vi "Read Limit Test.vi"(0 "VISA resource name":refnum<visa-resource-name>, 5 "Measurement Type (6: Phase Noise)":u16(ring)=6 items=["AM Noise"=1, "Baseband Noise"=2, "Freq/Power"=3, "Spectrum"=4, "Transient"=5, "Phase Noise"=6, "User"=7], 11 "error in (no error)":errorcluster, 12 "Maximum Time (10000 ms)":u32=10000) -> (1 "Trace 1 Result":enum16{"Pass", "Fail", ""}(ring)=enum."", 2 "Trace 2 Result":enum16{"Pass", "Fail", ""}(ring)=enum."", 3 "Trace 3 Result":enum16{"Pass", "Fail", ""}(ring)=enum."", 4 "VISA resource name out":refnum<visa-resource-name>, 6 "Trace 4 Result":enum16{"Pass", "Fail", ""}(ring)=enum."", 8 "Trace 5 Result":enum16{"Pass", "Fail", ""}(ring)=enum."", 10 "Trace 6 Result":enum16{"Pass", "Fail", ""}(ring)=enum."", 13 "Trace 8 Result":enum16{"Pass", "Fail", ""}(ring)=enum."", 14 "Trace 7 Result":enum16{"Pass", "Fail", ""}(ring)=enum."", 15 "error out":errorcluster)   [LabVIEW 2011, in "Agilent E5052X.lvlib"]
doc: "Reads the limit line test results for all traces and all kinds of measurements.\n\n<b>Note: </b> \n\nUse the \"Clear-Load Limit Line\" utility VI to load a user specified limit line. Use the \"Configure Limit Test\" VI to enable the limit line and change other settings. If \"Enable Limit Line\" control in the \"Configure Limit Test\" VI is not enabled, the test will always pass."
uses:
  Agilent E5052X.lvlib
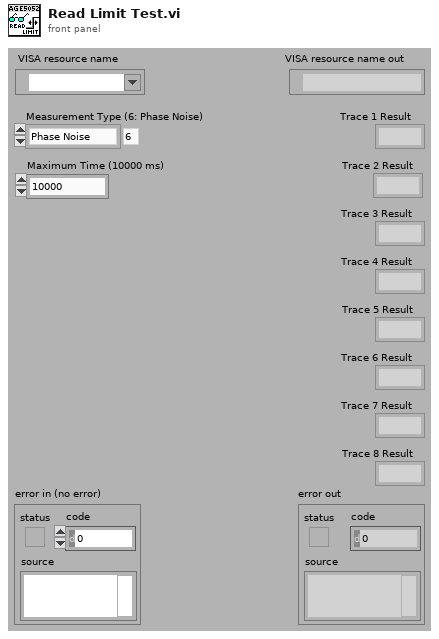
[diagram p1: front panel]
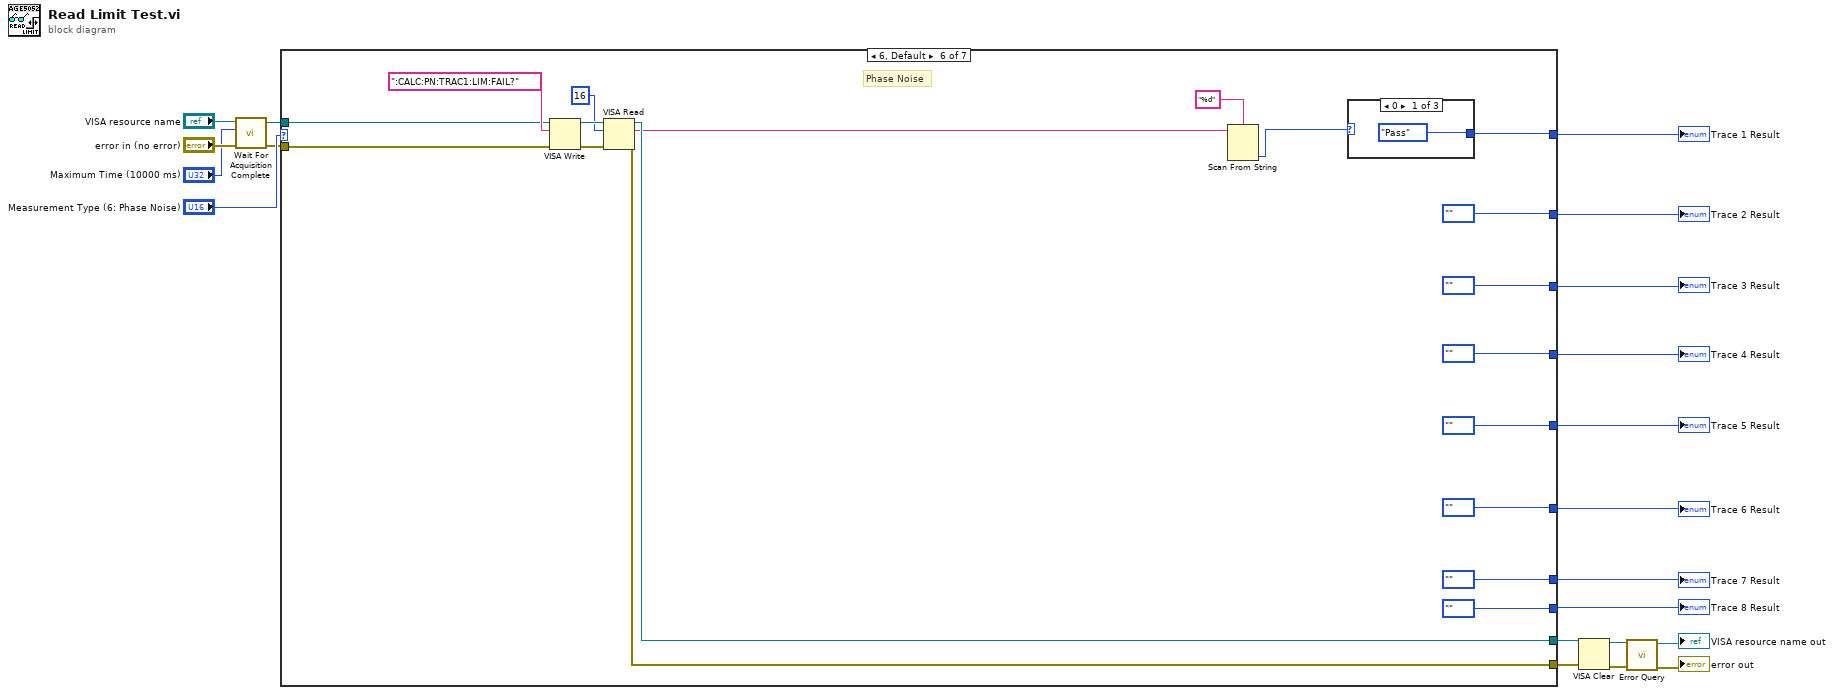
[diagram p0: block diagram]
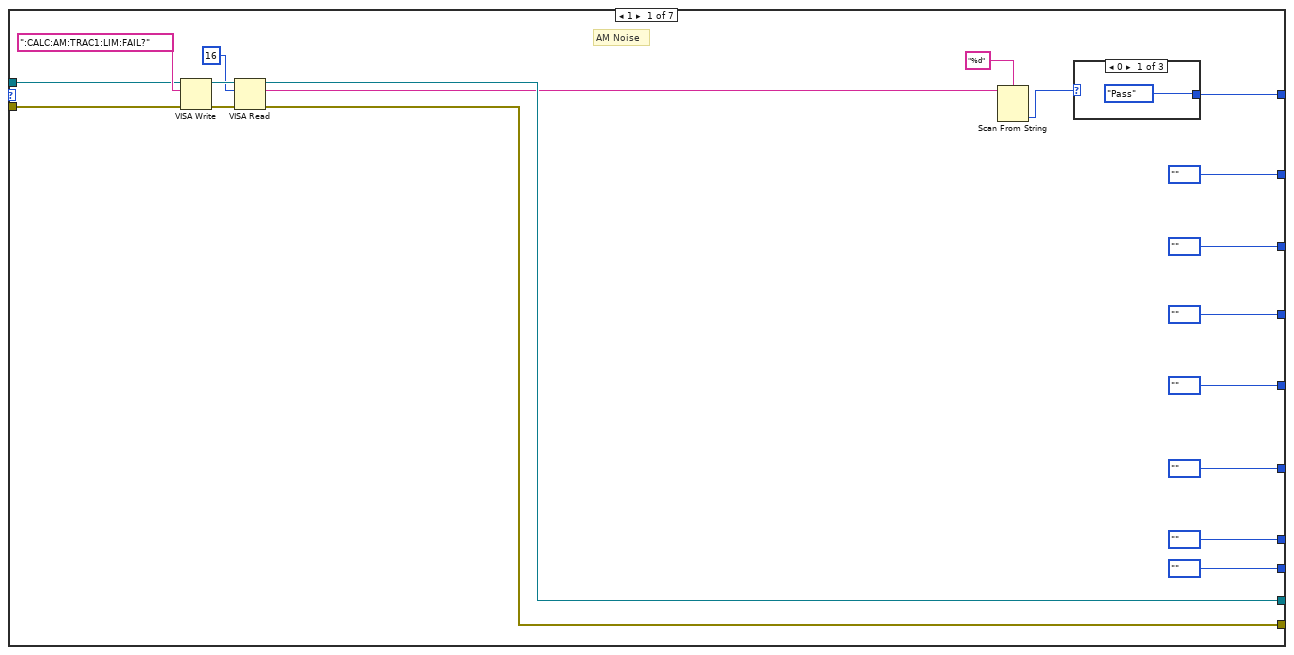
[diagram p2: hidden frame]
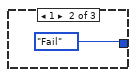
[diagram p3: hidden frame]
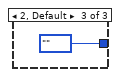
[diagram p4: hidden frame]
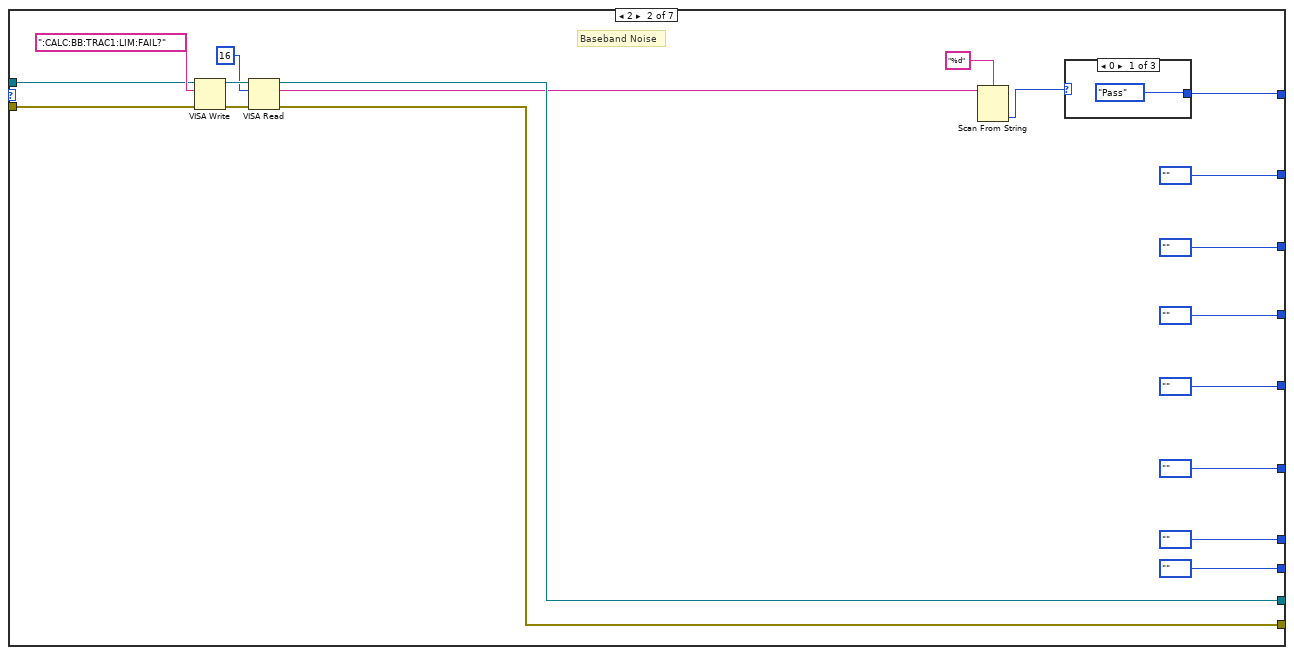
[diagram p5: hidden frame]
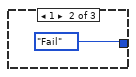
[diagram p6: hidden frame]
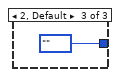
[diagram p7: hidden frame]
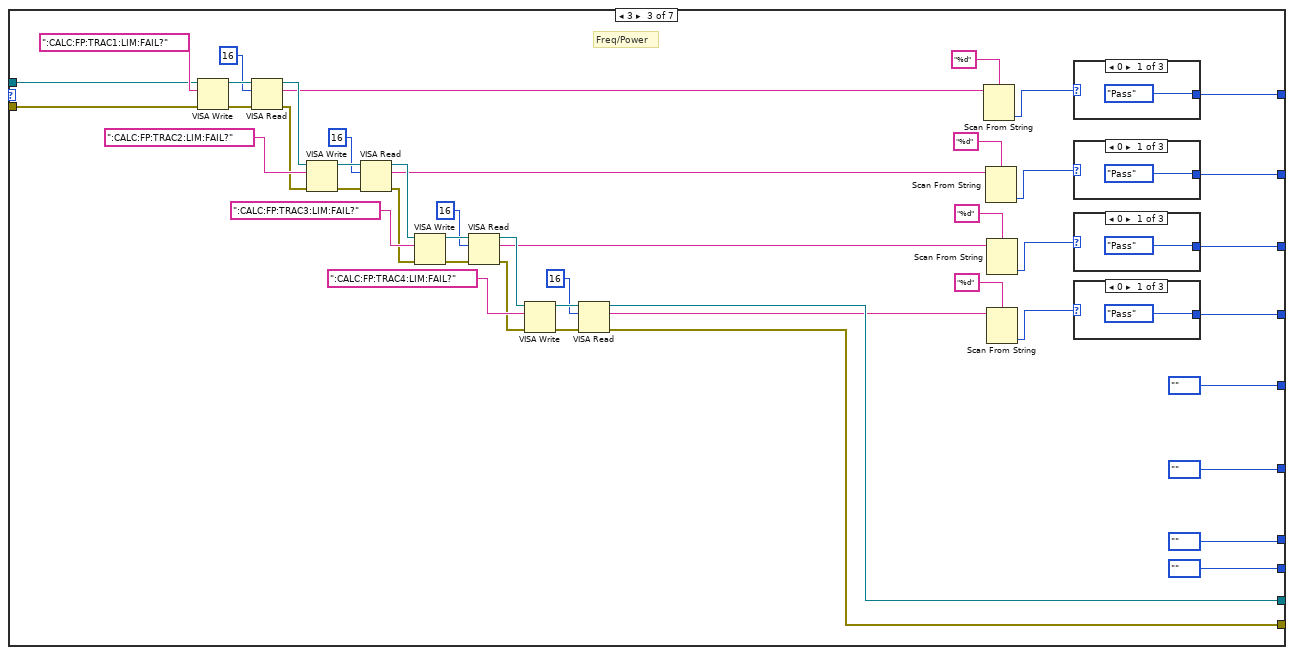
[diagram p8: hidden frame]
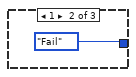
[diagram p9: hidden frame]
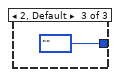
[diagram p10: hidden frame]
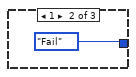
[diagram p11: hidden frame]
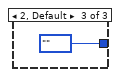
[diagram p12: hidden frame]
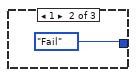
[diagram p13: hidden frame]
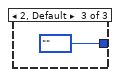
[diagram p14: hidden frame]
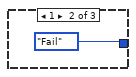
[diagram p15: hidden frame]
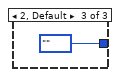
[diagram p16: hidden frame]
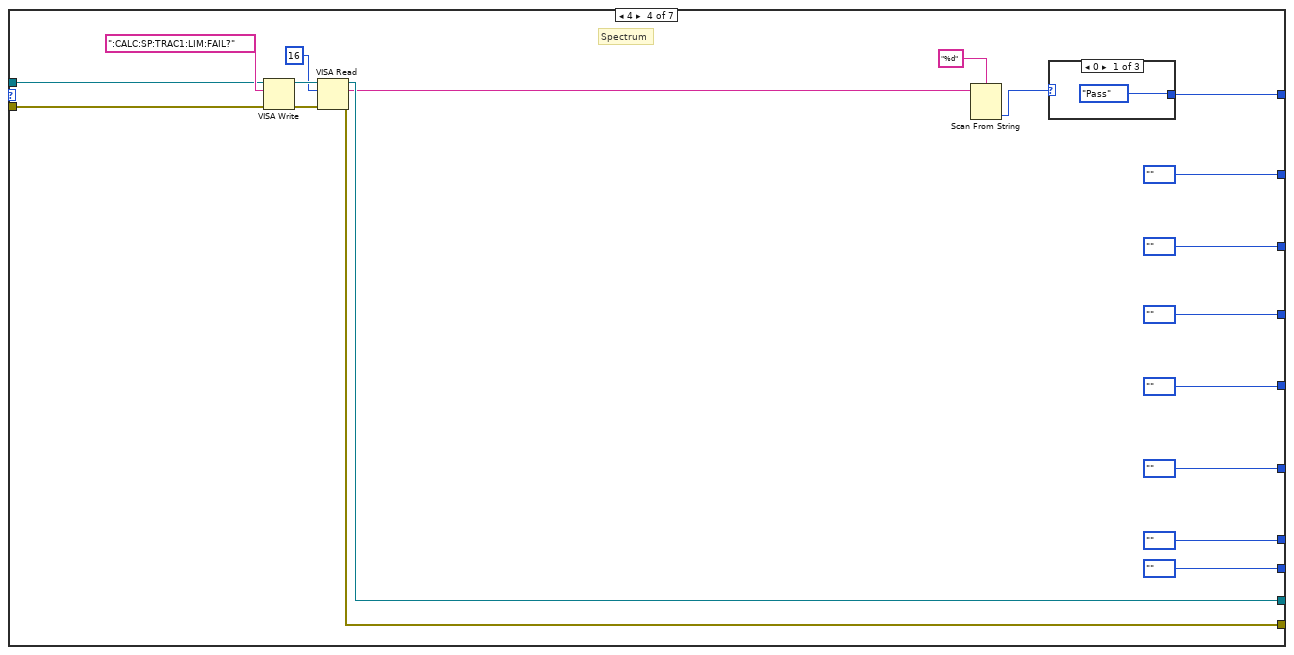
[diagram p17: hidden frame]
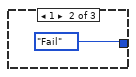
[diagram p18: hidden frame]
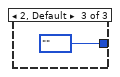
[diagram p19: hidden frame]
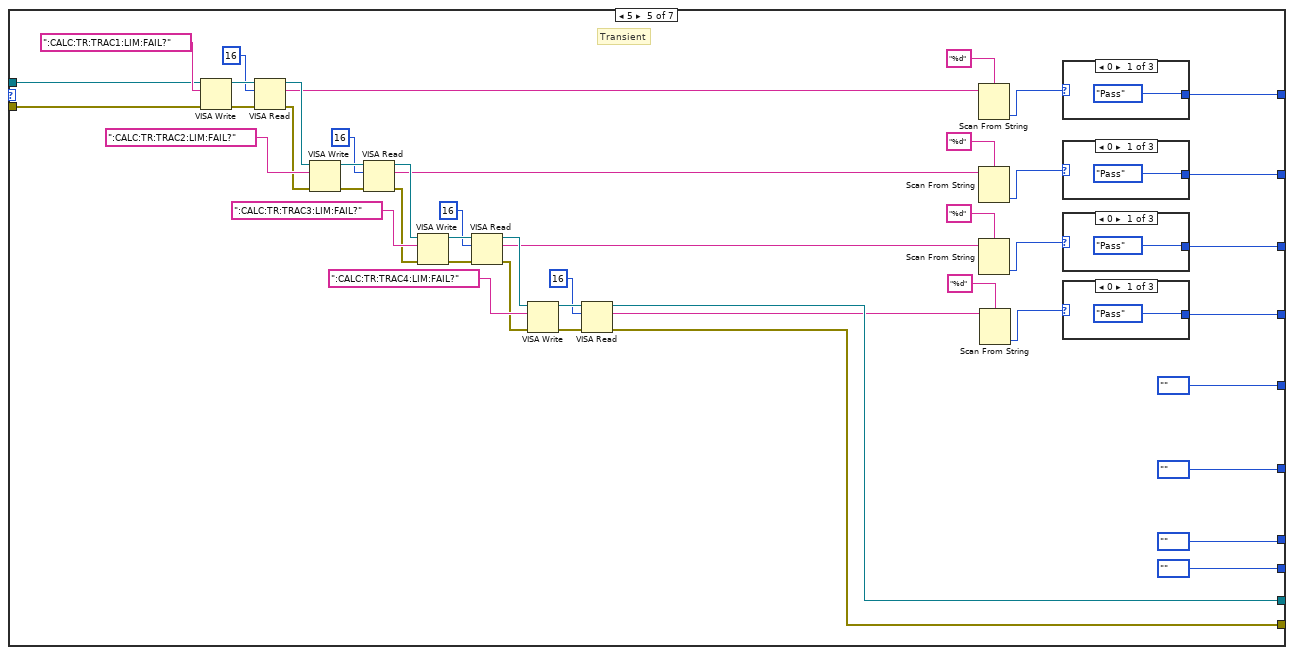
[diagram p20: hidden frame]
diagram:
  n1 = call "Wait For Acquisition Complete.vi"("error in (no error)"="error in (no error)", "Maximum Time (10000)"="Maximum Time (10000 ms)", "VISA resource name"="VISA resource name") -> ("error out"=w6:errorcluster, "VISA resource name out"=w7:refnum<visa-resource-name>)  [unwired: 7 in]
  n2 = case shown="6, Default" "Measurement Type (6: Phase Noise)" {
    tunnel: w7 -> [w35 w57 w106 w137 w168 w217 w284]
    tunnel: w6 -> [w34 w56 w105 w136 w167 w216 w283]
    tunnel: [w33 w55 w86 w135 w166 w215 w258] -> w12
    tunnel: [w32 w54 w85 w134 w165 w214 w257] -> w11
    tunnel: [w31 w53 w84 w133 w164 w213 w256] -> w20
    tunnel: [enum16{"Pass", "Fail", ""}."" ("Trace 1 Result") enum16{"Pass", "Fail", ""}."" ("Trace 1 Result") w83 enum16{"Pass", "Fail", ""}."" ("Trace 1 Result") w163 enum16{"Pass", "Fail", ""}."" ("Trace 1 Result") w255] -> w19
    tunnel: [enum16{"Pass", "Fail", ""}."" ("Trace 1 Result") enum16{"Pass", "Fail", ""}."" ("Trace 1 Result") w82 enum16{"Pass", "Fail", ""}."" ("Trace 1 Result") w162 enum16{"Pass", "Fail", ""}."" ("Trace 1 Result") w254] -> w18
    tunnel: [enum16{"Pass", "Fail", ""}."" ("Trace 1 Result") enum16{"Pass", "Fail", ""}."" ("Trace 1 Result") w81 enum16{"Pass", "Fail", ""}."" ("Trace 1 Result") w161 enum16{"Pass", "Fail", ""}."" ("Trace 1 Result") w253] -> w17
    tunnel: [enum16{"Pass", "Fail", ""}."" ("Trace 1 Result") enum16{"Pass", "Fail", ""}."" ("Trace 1 Result") enum16{"Pass", "Fail", ""}."" ("Trace 1 Result") enum16{"Pass", "Fail", ""}."" ("Trace 1 Result") enum16{"Pass", "Fail", ""}."" ("Trace 1 Result") enum16{"Pass", "Fail", ""}."" ("Trace 1 Result") w249] -> w16
    tunnel: [enum16{"Pass", "Fail", ""}."" ("Trace 1 Result") enum16{"Pass", "Fail", ""}."" ("Trace 1 Result") enum16{"Pass", "Fail", ""}."" ("Trace 1 Result") enum16{"Pass", "Fail", ""}."" ("Trace 1 Result") enum16{"Pass", "Fail", ""}."" ("Trace 1 Result") enum16{"Pass", "Fail", ""}."" ("Trace 1 Result") w250] -> w15
    tunnel: [enum16{"Pass", "Fail", ""}."" ("Trace 1 Result") enum16{"Pass", "Fail", ""}."" ("Trace 1 Result") enum16{"Pass", "Fail", ""}."" ("Trace 1 Result") enum16{"Pass", "Fail", ""}."" ("Trace 1 Result") enum16{"Pass", "Fail", ""}."" ("Trace 1 Result") enum16{"Pass", "Fail", ""}."" ("Trace 1 Result") w251] -> w14
    tunnel: [enum16{"Pass", "Fail", ""}."" ("Trace 1 Result") enum16{"Pass", "Fail", ""}."" ("Trace 1 Result") enum16{"Pass", "Fail", ""}."" ("Trace 1 Result") enum16{"Pass", "Fail", ""}."" ("Trace 1 Result") enum16{"Pass", "Fail", ""}."" ("Trace 1 Result") enum16{"Pass", "Fail", ""}."" ("Trace 1 Result") w252] -> w13
    frame 1 {
      # "AM Noise"
      n3 = VISA Write(VISA resource name=w35, write buffer=":CALC:AM:TRAC1:LIM:FAIL?", error in (no error)=w34) -> (VISA resource name out=w37:refnum<visa-resource-name>, error out=w38:errorcluster)  [unwired: 1 out]
      n4 = VISA Read(VISA resource name=w37, byte count=u32 16, error in (no error)=w38) -> (VISA resource name out=w33:refnum<visa-resource-name>, read buffer=w22:string, error out=w32:errorcluster)  [unwired: 1 out]
      n5 = Scan From String(format string="%d", input string=w22) -> (output 1=w21:i32)  [unwired: 3 in, 3 out]
      n6 = case shown="0" w21 {
        tunnel: [enum16{"Pass", "Fail", ""}."Pass" ("Trace 1 Result") enum16{"Pass", "Fail", ""}."Fail" ("Trace 1 Result") enum16{"Pass", "Fail", ""}."" ("Trace 1 Result")] -> w31
        frame 0 {
        }
        frame 1 {
        }
        frame 2, Default {
        }
      }
    }
    frame 2 {
      # "Baseband Noise"
      n7 = VISA Write(VISA resource name=w57, write buffer=":CALC:BB:TRAC1:LIM:FAIL?", error in (no error)=w56) -> (VISA resource name out=w59:refnum<visa-resource-name>, error out=w60:errorcluster)  [unwired: 1 out]
      n8 = VISA Read(VISA resource name=w59, byte count=u32 16, error in (no error)=w60) -> (VISA resource name out=w55:refnum<visa-resource-name>, read buffer=w44:string, error out=w54:errorcluster)  [unwired: 1 out]
      n9 = Scan From String(format string="%d", input string=w44) -> (output 1=w43:i32)  [unwired: 3 in, 3 out]
      n10 = case shown="0" w43 {
        tunnel: [enum16{"Pass", "Fail", ""}."Pass" ("Trace 1 Result") enum16{"Pass", "Fail", ""}."Fail" ("Trace 1 Result") enum16{"Pass", "Fail", ""}."" ("Trace 1 Result")] -> w53
        frame 0 {
        }
        frame 1 {
        }
        frame 2, Default {
        }
      }
    }
    frame 3 {
      # "Freq/Power"
      n11 = VISA Write(VISA resource name=w106, write buffer=":CALC:FP:TRAC1:LIM:FAIL?", error in (no error)=w105) -> (VISA resource name out=w108:refnum<visa-resource-name>, error out=w109:errorcluster)  [unwired: 1 out]
      n12 = VISA Read(VISA resource name=w108, byte count=u32 16, error in (no error)=w109) -> (VISA resource name out=w99:refnum<visa-resource-name>, read buffer=w75:string, error out=w100:errorcluster)  [unwired: 1 out]
      n13 = VISA Write(VISA resource name=w99, write buffer=":CALC:FP:TRAC2:LIM:FAIL?", error in (no error)=w100) -> (VISA resource name out=w102:refnum<visa-resource-name>, error out=w103:errorcluster)  [unwired: 1 out]
      n14 = VISA Read(VISA resource name=w102, byte count=u32 16, error in (no error)=w103) -> (VISA resource name out=w93:refnum<visa-resource-name>, read buffer=w72:string, error out=w94:errorcluster)  [unwired: 1 out]
      n15 = VISA Write(VISA resource name=w93, write buffer=":CALC:FP:TRAC3:LIM:FAIL?", error in (no error)=w94) -> (VISA resource name out=w96:refnum<visa-resource-name>, error out=w97:errorcluster)  [unwired: 1 out]
      n16 = VISA Read(VISA resource name=w96, byte count=u32 16, error in (no error)=w97) -> (VISA resource name out=w87:refnum<visa-resource-name>, read buffer=w69:string, error out=w88:errorcluster)  [unwired: 1 out]
      n17 = VISA Write(VISA resource name=w87, write buffer=":CALC:FP:TRAC4:LIM:FAIL?", error in (no error)=w88) -> (VISA resource name out=w90:refnum<visa-resource-name>, error out=w91:errorcluster)  [unwired: 1 out]
      n18 = VISA Read(VISA resource name=w90, byte count=u32 16, error in (no error)=w91) -> (VISA resource name out=w86:refnum<visa-resource-name>, read buffer=w66:string, error out=w85:errorcluster)  [unwired: 1 out]
      n19 = Scan From String(format string="%d", input string=w75) -> (output 1=w74:i32)  [unwired: 3 in, 3 out]
      n20 = Scan From String(format string="%d", input string=w72) -> (output 1=w71:i32)  [unwired: 3 in, 3 out]
      n21 = Scan From String(format string="%d", input string=w69) -> (output 1=w68:i32)  [unwired: 3 in, 3 out]
      n22 = Scan From String(format string="%d", input string=w66) -> (output 1=w65:i32)  [unwired: 3 in, 3 out]
      n23 = case shown="0" w74 {
        tunnel: [enum16{"Pass", "Fail", ""}."Pass" ("Trace 1 Result") enum16{"Pass", "Fail", ""}."Fail" ("Trace 1 Result") enum16{"Pass", "Fail", ""}."" ("Trace 1 Result")] -> w84
        frame 0 {
        }
        frame 1 {
        }
        frame 2, Default {
        }
      }
      n24 = case shown="0" w71 {
        tunnel: [enum16{"Pass", "Fail", ""}."Pass" ("Trace 1 Result") enum16{"Pass", "Fail", ""}."Fail" ("Trace 1 Result") enum16{"Pass", "Fail", ""}."" ("Trace 1 Result")] -> w83
        frame 0 {
        }
        frame 1 {
        }
        frame 2, Default {
        }
      }
      n25 = case shown="0" w68 {
        tunnel: [enum16{"Pass", "Fail", ""}."Pass" ("Trace 1 Result") enum16{"Pass", "Fail", ""}."Fail" ("Trace 1 Result") enum16{"Pass", "Fail", ""}."" ("Trace 1 Result")] -> w82
        frame 0 {
        }
        frame 1 {
        }
        frame 2, Default {
        }
      }
      n26 = case shown="0" w65 {
        tunnel: [enum16{"Pass", "Fail", ""}."Pass" ("Trace 1 Result") enum16{"Pass", "Fail", ""}."Fail" ("Trace 1 Result") enum16{"Pass", "Fail", ""}."" ("Trace 1 Result")] -> w81
        frame 0 {
        }
        frame 1 {
        }
        frame 2, Default {
        }
      }
    }
    frame 4 {
      # "Spectrum"
      n27 = VISA Write(VISA resource name=w137, write buffer=":CALC:SP:TRAC1:LIM:FAIL?", error in (no error)=w136) -> (VISA resource name out=w139:refnum<visa-resource-name>, error out=w140:errorcluster)  [unwired: 1 out]
      n28 = VISA Read(VISA resource name=w139, byte count=u32 16, error in (no error)=w140) -> (VISA resource name out=w135:refnum<visa-resource-name>, read buffer=w124:string, error out=w134:errorcluster)  [unwired: 1 out]
      n29 = Scan From String(format string="%d", input string=w124) -> (output 1=w123:i32)  [unwired: 3 in, 3 out]
      n30 = case shown="0" w123 {
        tunnel: [enum16{"Pass", "Fail", ""}."Pass" ("Trace 1 Result") enum16{"Pass", "Fail", ""}."Fail" ("Trace 1 Result") enum16{"Pass", "Fail", ""}."" ("Trace 1 Result")] -> w133
        frame 0 {
        }
        frame 1 {
        }
        frame 2, Default {
        }
      }
    }
    frame 5 {
      # "Transient"
      n31 = VISA Write(VISA resource name=w168, write buffer=":CALC:TR:TRAC1:LIM:FAIL?", error in (no error)=w167) -> (VISA resource name out=w188:refnum<visa-resource-name>, error out=w189:errorcluster)  [unwired: 1 out]
      n32 = VISA Read(VISA resource name=w188, byte count=u32 16, error in (no error)=w189) -> (VISA resource name out=w181:refnum<visa-resource-name>, read buffer=w155:string, error out=w182:errorcluster)  [unwired: 1 out]
      n33 = VISA Write(VISA resource name=w181, write buffer=":CALC:TR:TRAC2:LIM:FAIL?", error in (no error)=w182) -> (VISA resource name out=w184:refnum<visa-resource-name>, error out=w185:errorcluster)  [unwired: 1 out]
      n34 = VISA Read(VISA resource name=w184, byte count=u32 16, error in (no error)=w185) -> (VISA resource name out=w175:refnum<visa-resource-name>, read buffer=w152:string, error out=w176:errorcluster)  [unwired: 1 out]
      n35 = VISA Write(VISA resource name=w175, write buffer=":CALC:TR:TRAC3:LIM:FAIL?", error in (no error)=w176) -> (VISA resource name out=w178:refnum<visa-resource-name>, error out=w179:errorcluster)  [unwired: 1 out]
      n36 = VISA Read(VISA resource name=w178, byte count=u32 16, error in (no error)=w179) -> (VISA resource name out=w169:refnum<visa-resource-name>, read buffer=w149:string, error out=w170:errorcluster)  [unwired: 1 out]
      n37 = VISA Write(VISA resource name=w169, write buffer=":CALC:TR:TRAC4:LIM:FAIL?", error in (no error)=w170) -> (VISA resource name out=w172:refnum<visa-resource-name>, error out=w173:errorcluster)  [unwired: 1 out]
      n38 = VISA Read(VISA resource name=w172, byte count=u32 16, error in (no error)=w173) -> (VISA resource name out=w166:refnum<visa-resource-name>, read buffer=w146:string, error out=w165:errorcluster)  [unwired: 1 out]
      n39 = Scan From String(format string="%d", input string=w155) -> (output 1=w154:i32)  [unwired: 3 in, 3 out]
      n40 = Scan From String(format string="%d", input string=w152) -> (output 1=w151:i32)  [unwired: 3 in, 3 out]
      n41 = Scan From String(format string="%d", input string=w149) -> (output 1=w148:i32)  [unwired: 3 in, 3 out]
      n42 = Scan From String(format string="%d", input string=w146) -> (output 1=w145:i32)  [unwired: 3 in, 3 out]
      n43 = case shown="0" w154 {
        tunnel: [enum16{"Pass", "Fail", ""}."Pass" ("Trace 1 Result") enum16{"Pass", "Fail", ""}."Fail" ("Trace 1 Result") enum16{"Pass", "Fail", ""}."" ("Trace 1 Result")] -> w164
        frame 0 {
        }
        frame 1 {
        }
        frame 2, Default {
        }
      }
      n44 = case shown="0" w151 {
        tunnel: [enum16{"Pass", "Fail", ""}."Pass" ("Trace 1 Result") enum16{"Pass", "Fail", ""}."Fail" ("Trace 1 Result") enum16{"Pass", "Fail", ""}."" ("Trace 1 Result")] -> w163
        frame 0 {
        }
        frame 1 {
        }
        frame 2, Default {
        }
      }
      n45 = case shown="0" w148 {
        tunnel: [enum16{"Pass", "Fail", ""}."Pass" ("Trace 1 Result") enum16{"Pass", "Fail", ""}."Fail" ("Trace 1 Result") enum16{"Pass", "Fail", ""}."" ("Trace 1 Result")] -> w162
        frame 0 {
        }
        frame 1 {
        }
        frame 2, Default {
        }
      }
      n46 = case shown="0" w145 {
        tunnel: [enum16{"Pass", "Fail", ""}."Pass" ("Trace 1 Result") enum16{"Pass", "Fail", ""}."Fail" ("Trace 1 Result") enum16{"Pass", "Fail", ""}."" ("Trace 1 Result")] -> w161
        frame 0 {
        }
        frame 1 {
        }
        frame 2, Default {
        }
      }
    }
    frame 6, Default {
      # "Phase Noise"
      n47 = VISA Write(VISA resource name=w217, write buffer=":CALC:PN:TRAC1:LIM:FAIL?", error in (no error)=w216) -> (VISA resource name out=w219:refnum<visa-resource-name>, error out=w220:errorcluster)  [unwired: 1 out]
      n48 = VISA Read(VISA resource name=w219, byte count=u32 16, error in (no error)=w220) -> (VISA resource name out=w215:refnum<visa-resource-name>, read buffer=w205:string, error out=w214:errorcluster)  [unwired: 1 out]
      n49 = Scan From String(format string="%d", input string=w205) -> (output 1=w203:i32)  [unwired: 3 in, 3 out]
      n50 = case shown="0" w203 {
        tunnel: [enum16{"Pass", "Fail", ""}."Pass" ("Trace 1 Result") enum16{"Pass", "Fail", ""}."Fail" ("Trace 1 Result") enum16{"Pass", "Fail", ""}."" ("Trace 1 Result")] -> w213
        frame 0 {
        }
        frame 1 {
        }
        frame 2, Default {
        }
      }
    }
    frame 7 {
      # "User"
      n51 = VISA Write(VISA resource name=w284, write buffer=":CALC:USER:TRAC1:LIM:FAIL?", error in (no error)=w283) -> (VISA resource name out=w304:refnum<visa-resource-name>, error out=w305:errorcluster)  [unwired: 1 out]
      n52 = VISA Read(VISA resource name=w304, byte count=u32 16, error in (no error)=w305) -> (VISA resource name out=w297:refnum<visa-resource-name>, read buffer=w247:string, error out=w298:errorcluster)  [unwired: 1 out]
      n53 = VISA Write(VISA resource name=w297, write buffer=":CALC:USER:TRAC2:LIM:FAIL?", error in (no error)=w298) -> (VISA resource name out=w300:refnum<visa-resource-name>, error out=w301:errorcluster)  [unwired: 1 out]
      n54 = VISA Read(VISA resource name=w300, byte count=u32 16, error in (no error)=w301) -> (VISA resource name out=w291:refnum<visa-resource-name>, read buffer=w244:string, error out=w292:errorcluster)  [unwired: 1 out]
      n55 = VISA Write(VISA resource name=w291, write buffer=":CALC:USER:TRAC3:LIM:FAIL?", error in (no error)=w292) -> (VISA resource name out=w294:refnum<visa-resource-name>, error out=w295:errorcluster)  [unwired: 1 out]
      n56 = VISA Read(VISA resource name=w294, byte count=u32 16, error in (no error)=w295) -> (VISA resource name out=w285:refnum<visa-resource-name>, read buffer=w241:string, error out=w286:errorcluster)  [unwired: 1 out]
      n57 = VISA Write(VISA resource name=w285, write buffer=":CALC:USER:TRAC4:LIM:FAIL?", error in (no error)=w286) -> (VISA resource name out=w288:refnum<visa-resource-name>, error out=w289:errorcluster)  [unwired: 1 out]
      n58 = VISA Read(VISA resource name=w288, byte count=u32 16, error in (no error)=w289) -> (VISA resource name out=w259:refnum<visa-resource-name>, read buffer=w238:string, error out=w260:errorcluster)  [unwired: 1 out]
      n59 = VISA Write(VISA resource name=w259, write buffer=":CALC:USER:TRAC5:LIM:FAIL?", error in (no error)=w260) -> (VISA resource name out=w280:refnum<visa-resource-name>, error out=w281:errorcluster)  [unwired: 1 out]
      n60 = VISA Read(VISA resource name=w280, byte count=u32 16, error in (no error)=w281) -> (VISA resource name out=w273:refnum<visa-resource-name>, read buffer=w235:string, error out=w274:errorcluster)  [unwired: 1 out]
      n61 = VISA Write(VISA resource name=w273, write buffer=":CALC:USER:TRAC6:LIM:FAIL?", error in (no error)=w274) -> (VISA resource name out=w276:refnum<visa-resource-name>, error out=w277:errorcluster)  [unwired: 1 out]
      n62 = VISA Read(VISA resource name=w276, byte count=u32 16, error in (no error)=w277) -> (VISA resource name out=w267:refnum<visa-resource-name>, read buffer=w232:string, error out=w268:errorcluster)  [unwired: 1 out]
      n63 = Scan From String(format string="%d", input string=w244) -> (output 1=w243:i32)  [unwired: 3 in, 3 out]
      n64 = Scan From String(format string="%d", input string=w247) -> (output 1=w246:i32)  [unwired: 3 in, 3 out]
      n65 = Scan From String(format string="%d", input string=w241) -> (output 1=w240:i32)  [unwired: 3 in, 3 out]
      n66 = Scan From String(format string="%d", input string=w238) -> (output 1=w237:i32)  [unwired: 3 in, 3 out]
      n67 = VISA Write(VISA resource name=w267, write buffer=":CALC:USER:TRAC7:LIM:FAIL?", error in (no error)=w268) -> (VISA resource name out=w270:refnum<visa-resource-name>, error out=w271:errorcluster)  [unwired: 1 out]
      n68 = case shown="0" w246 {
        tunnel: [enum16{"Pass", "Fail", ""}."Pass" ("Trace 1 Result") enum16{"Pass", "Fail", ""}."Fail" ("Trace 1 Result") enum16{"Pass", "Fail", ""}."" ("Trace 1 Result")] -> w256
        frame 0 {
        }
        frame 1 {
        }
        frame 2, Default {
        }
      }
      n69 = case shown="0" w243 {
        tunnel: [enum16{"Pass", "Fail", ""}."Pass" ("Trace 1 Result") enum16{"Pass", "Fail", ""}."Fail" ("Trace 1 Result") enum16{"Pass", "Fail", ""}."" ("Trace 1 Result")] -> w255
        frame 0 {
        }
        frame 1 {
        }
        frame 2, Default {
        }
      }
      n70 = case shown="0" w240 {
        tunnel: [enum16{"Pass", "Fail", ""}."Pass" ("Trace 1 Result") enum16{"Pass", "Fail", ""}."Fail" ("Trace 1 Result") enum16{"Pass", "Fail", ""}."" ("Trace 1 Result")] -> w254
        frame 0 {
        }
        frame 1 {
        }
        frame 2, Default {
        }
      }
      n71 = case shown="0" w237 {
        tunnel: [enum16{"Pass", "Fail", ""}."Pass" ("Trace 1 Result") enum16{"Pass", "Fail", ""}."Fail" ("Trace 1 Result") enum16{"Pass", "Fail", ""}."" ("Trace 1 Result")] -> w253
        frame 0 {
        }
        frame 1 {
        }
        frame 2, Default {
        }
      }
      n72 = VISA Read(VISA resource name=w270, byte count=u32 16, error in (no error)=w271) -> (VISA resource name out=w261:refnum<visa-resource-name>, read buffer=w229:string, error out=w262:errorcluster)  [unwired: 1 out]
      n73 = VISA Write(VISA resource name=w261, write buffer=":CALC:USER:TRAC8:LIM:FAIL?", error in (no error)=w262) -> (VISA resource name out=w264:refnum<visa-resource-name>, error out=w265:errorcluster)  [unwired: 1 out]
      n74 = VISA Read(VISA resource name=w264, byte count=u32 16, error in (no error)=w265) -> (VISA resource name out=w258:refnum<visa-resource-name>, read buffer=w226:string, error out=w257:errorcluster)  [unwired: 1 out]
      n75 = Scan From String(format string="%d", input string=w226) -> (output 1=w225:i32)  [unwired: 3 in, 3 out]
      n76 = Scan From String(format string="%d", input string=w235) -> (output 1=w234:i32)  [unwired: 3 in, 3 out]
      n77 = Scan From String(format string="%d", input string=w232) -> (output 1=w231:i32)  [unwired: 3 in, 3 out]
      n78 = Scan From String(format string="%d", input string=w229) -> (output 1=w228:i32)  [unwired: 3 in, 3 out]
      n79 = case shown="0" w234 {
        tunnel: [enum16{"Pass", "Fail", ""}."Pass" ("Trace 1 Result") enum16{"Pass", "Fail", ""}."Fail" ("Trace 1 Result") enum16{"Pass", "Fail", ""}."" ("Trace 1 Result")] -> w249
        frame 0 {
        }
        frame 1 {
        }
        frame 2, Default {
        }
      }
      n80 = case shown="0" w231 {
        tunnel: [enum16{"Pass", "Fail", ""}."Pass" ("Trace 1 Result") enum16{"Pass", "Fail", ""}."Fail" ("Trace 1 Result") enum16{"Pass", "Fail", ""}."" ("Trace 1 Result")] -> w250
        frame 0 {
        }
        frame 1 {
        }
        frame 2, Default {
        }
      }
      n81 = case shown="0" w228 {
        tunnel: [enum16{"Pass", "Fail", ""}."Pass" ("Trace 1 Result") enum16{"Pass", "Fail", ""}."Fail" ("Trace 1 Result") enum16{"Pass", "Fail", ""}."" ("Trace 1 Result")] -> w251
        frame 0 {
        }
        frame 1 {
        }
        frame 2, Default {
        }
      }
      n82 = case shown="0" w225 {
        tunnel: [enum16{"Pass", "Fail", ""}."Pass" ("Trace 1 Result") enum16{"Pass", "Fail", ""}."Fail" ("Trace 1 Result") enum16{"Pass", "Fail", ""}."" ("Trace 1 Result")] -> w252
        frame 0 {
        }
        frame 1 {
        }
        frame 2, Default {
        }
      }
    }
  }
  "Trace 1 Result" <- w20
  "Trace 2 Result" <- w19
  "Trace 3 Result" <- w18
  "Trace 4 Result" <- w17
  "Trace 5 Result" <- w16
  "Trace 6 Result" <- w15
  "Trace 7 Result" <- w14
  "Trace 8 Result" <- w13
  n83 = VISA Clear(VISA resource name=w12, error in (no error)=w11) -> (VISA resource name out=w2:refnum<visa-resource-name>, error out=w1:errorcluster)
  n84 = call "Error Query.vi"("error in (no error)"=w1, "VISA resource name"=w2) -> ("error out"=→"error out":errorcluster, "VISA resource name out"=→"VISA resource name out":refnum<visa-resource-name>)  [unwired: 6 in, 2 out]
